vi "Loops ermitteln.vi"(8 "error in (no error)":errorcluster caption="Fehler (Eingang, kein Fehler)", 9 "PNS SprachIndex (Seite)":i32=24, 10 "Istwerte":u16[](array[numeric]), 11 "Steuerung PNS Eingang":refnum<class "Steuerung PNS.lvclass">) -> (0 "error out":errorcluster caption="Fehler (Ausgang)", 1 "Loopkennung":u16[](array[numeric]), 2 "Loops":string[](array[string]), 3 "Steuerung PNS Ausgang":refnum<class "Steuerung PNS.lvclass">)   [LabVIEW 2020, in "Steuerung PNS.lvclass"]
uses:
  Steuerung PNS.lvclass
  Sprachverwaltung/FGV Aktion Tabelle zerlegen.ctl
  Steuerung PNS.lvclass/Steuerung PNS.ctl
  Sprachverwaltung/Sprachverwaltung.lvlib
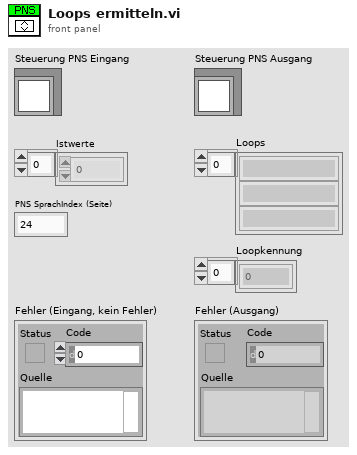
[diagram p1: front panel]
types:
  T1 = typedef "Sprachverwaltung.lvlib/FGV Aktion Tabelle zerlegen.ctl" = enum16{"laden", "vereinzeln", "speichern"}
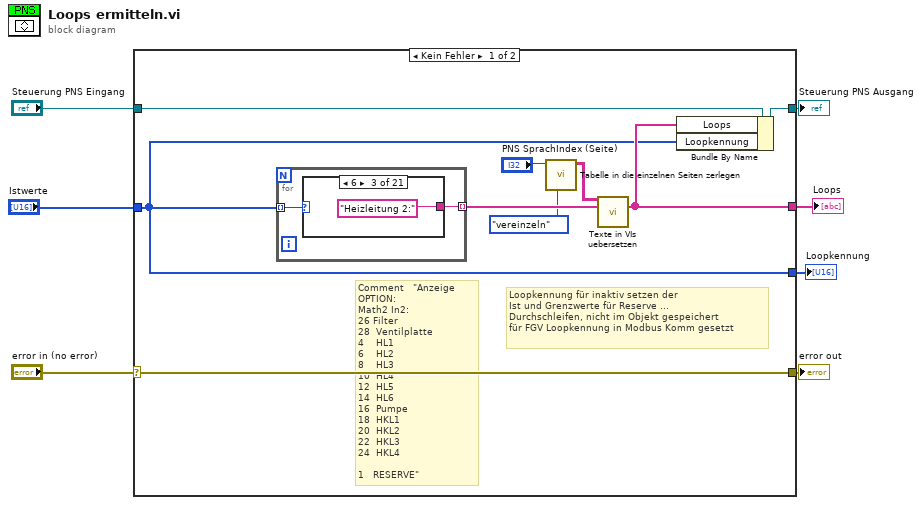
[diagram p0: block diagram]
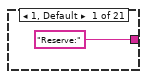
[diagram p2: hidden frame]
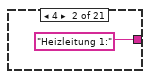
[diagram p3: hidden frame]
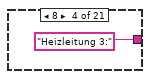
[diagram p4: hidden frame]
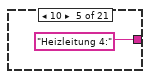
[diagram p5: hidden frame]
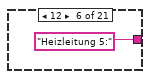
[diagram p6: hidden frame]
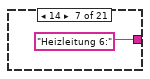
[diagram p7: hidden frame]
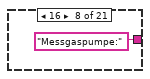
[diagram p8: hidden frame]
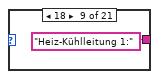
[diagram p9: hidden frame]
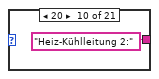
[diagram p10: hidden frame]
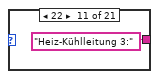
[diagram p11: hidden frame]
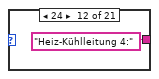
[diagram p12: hidden frame]
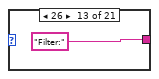
[diagram p13: hidden frame]
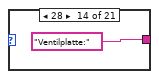
[diagram p14: hidden frame]
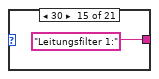
[diagram p15: hidden frame]
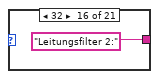
[diagram p16: hidden frame]
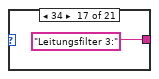
[diagram p17: hidden frame]
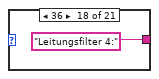
[diagram p18: hidden frame]
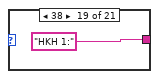
[diagram p19: hidden frame]
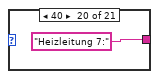
[diagram p20: hidden frame]
diagram:
  n1 = case shown="Kein Fehler" "error in (no error)" {
    selector: "error in (no error)" -> [w15 w43]
    tunnel: [w15 w43] -> w6
    tunnel: [w13 w42] -> w4
    tunnel: "Steuerung PNS Eingang" -> [w16 w42]
    tunnel: "Istwerte" -> [w10 _]
    tunnel: [w12 string[] [] ("String-Array zum Übersetzen")] -> w2
    tunnel: [w10 u16[] [] ("Istwerte")] -> w1
    frame No Error {
      # "Loopkennung für inaktiv setzen der \nIst und Grenzwerte für Reserve ...\nDurchschleifen, nicht im Objekt gespeichert\nfür FGV Loopkennung in Modbus Komm gesetzt"
      # "Comment\t\t\t\"Anzeige OPTION:\nMath2 In2:\n26 Filter\n28  Ventilplatte\n4    HL1\n6    HL2\n8    HL3\n10  HL4\n12  HL5\n14  HL6\n16  Pumpe\n18  HKL1\n20  HKL2\n22  HKL3\n24  HKL4\n\n1   RESERVE\""
      n2 = for {
        tunnel: w10 -> [w18] mode=indexing
        tunnel: [w17] -> w14 mode=indexing
        n3 = case shown="6" w18 {
          tunnel: ["Reserve:" "Heizleitung 1:" "Heizleitung 2:" "Heizleitung 3:" "Heizleitung 4:" "Heizleitung 5:" "Heizleitung 6:" "Messgaspumpe:" "Heiz-Kühlleitung 1:" "Heiz-Kühlleitung 2:" "Heiz-Kühlleitung 3:" "Heiz-Kühlleitung 4:" "Filter:" "Ventilplatte:" "Leitungsfilter 1:" "Leitungsfilter 2:" "Leitungsfilter 3:" "Leitungsfilter 4:" "HKH 1:" "Heizleitung 7:" "Heizleitung 8:"] -> w17
          frame 1, Default {
          }
          frame 4 {
          }
          frame 6 {
          }
          frame 8 {
          }
          frame 10 {
          }
          frame 12 {
          }
          frame 14 {
          }
          frame 16 {
          }
          frame 18 {
          }
          frame 20 {
          }
          frame 22 {
          }
          frame 24 {
          }
          frame 26 {
          }
          frame 28 {
          }
          frame 30 {
          }
          frame 32 {
          }
          frame 34 {
          }
          frame 36 {
          }
          frame 38 {
          }
          frame 40 {
          }
          frame 42 {
          }
        }
      }
      n4 = call "Tabelle in die einzelnen Seiten zerlegen.vi"("Aktion"=FGV_Aktion_Tabelle_zerlegen."vereinzeln", "Index (Seite)"="PNS SprachIndex (Seite)") -> ("Sprachliste"=w11:string[][])  [unwired: 7 in, 2 out]
      n5 = call "Texte in VIs uebersetzen.vi"("Sprachliste"=w11, "String-Array zum Übersetzen"=w14) -> ("String-Array zum Übersetzen"=w12:string[])  [unwired: 9 in, 4 out]
      n6 = Bundle By Name(cluster=w16, "Loops"=w12, "Loopkennung"=w10) -> (w13:refnum<class "Steuerung PNS.lvclass">)
    }
    frame Error {
    }
  }
  "error out" <- w6
  "Steuerung PNS Ausgang" <- w4
  "Loops" <- w2
  "Loopkennung" <- w1
